vi "FrictionComp_sub.vi"(6 "Vneg":dbl, 7 "Cneg":dbl, 9 "Cpos":dbl, 10 "Vpos":dbl, 11 "output y(t)":dbl) -> (3 "Numeric":dbl)   [LabVIEW 2021]
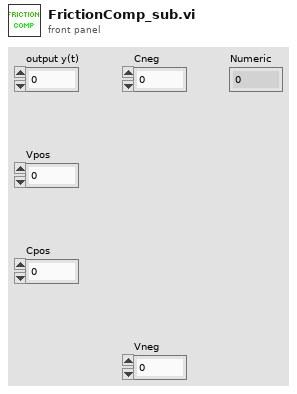
[diagram p1: front panel]
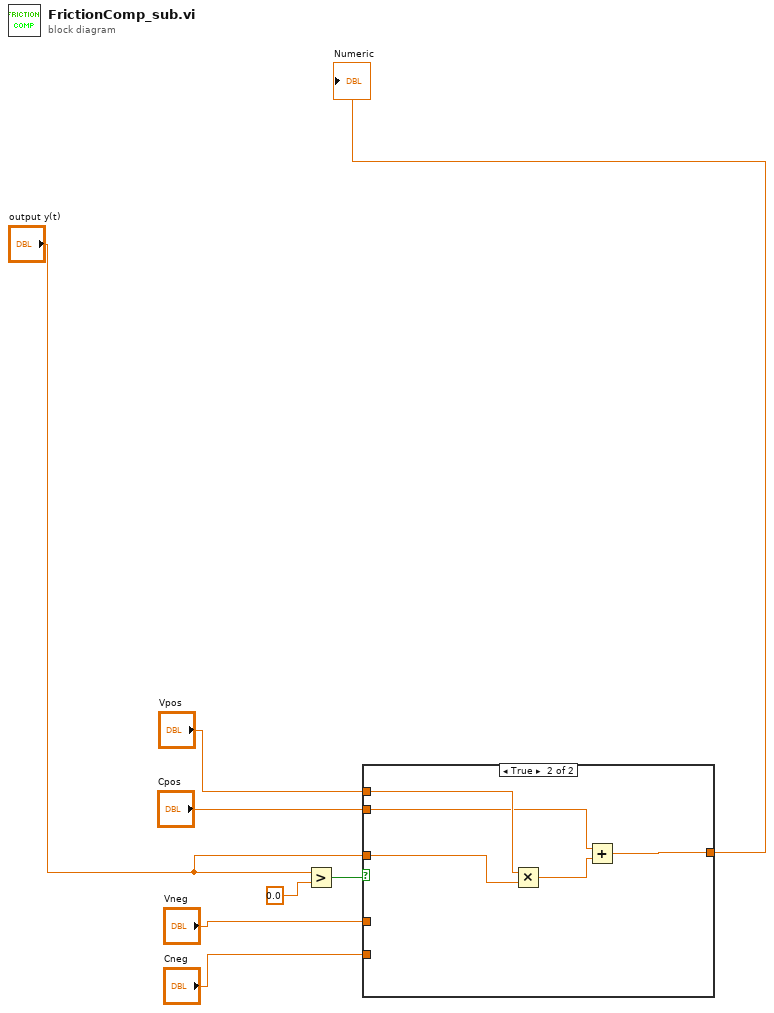
[diagram p0: block diagram]
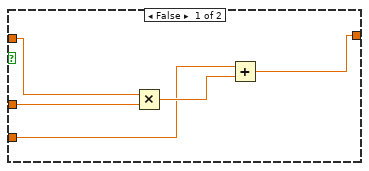
[diagram p2: hidden frame]
diagram:
  n1 = Greater?(x="output y(t)", y=0.0) -> (0:w2:bool)
  n2 = case shown="True" w2 {
    tunnel: [w9 w18] -> w1
    tunnel: "output y(t)" -> [w12 w17]
    tunnel: "Vpos" -> [_ w15]
    tunnel: "Cpos" -> [_ w14]
    tunnel: "Vneg" -> [w11 _]
    tunnel: "Cneg" -> [w10 _]
    frame False {
      n3 = Multiply ("Multiply 2")(x=w12, y=w11) -> (x*y=w13:dbl)
      n4 = Add ("Add 2")(x=w10, y=w13) -> (x+y=w9:dbl)
    }
    frame True {
      n5 = Multiply(x=w15, y=w17) -> (x*y=w16:dbl)
      n6 = Add(x=w14, y=w16) -> (x+y=w18:dbl)
    }
  }
  "Numeric" <- w1
